vi "EXTRACT-DATA-UINT32.vi"(2 "UINT32":u32, 7 "Data":u8[](array[numeric])) -> (4 "Value":u32, 8 "Min":u32, 10 "Max":u32, 15 "Inc":u32)   [LabVIEW 2011]
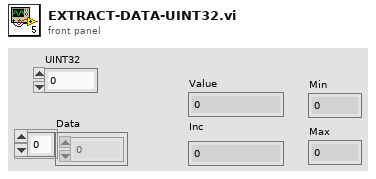
[diagram p1: front panel]
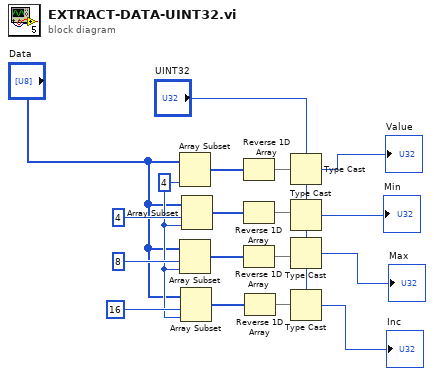
[diagram p0: block diagram]
diagram:
  w12 = 4 ("length")
  n1 = Array Subset(array="Data", length=w12) -> (w16:u8[])  [unwired: 1 in]
  n2 = Array Subset(array="Data", index=8, length=w12) -> (w17:u8[])
  n3 = Array Subset(array="Data", index=16, length=w12) -> (w11:u8[])
  n4 = Array Subset(array="Data", index=4, length=w12) -> (w18:u8[])
  n5 = Reverse 1D Array(array=w16) -> (reversed array=w10:u8[])
  n6 = Reverse 1D Array(array=w18) -> (reversed array=w9:u8[])
  n7 = Reverse 1D Array(array=w17) -> (reversed array=w8:u8[])
  n8 = Reverse 1D Array(array=w11) -> (reversed array=w7:u8[])
  n9 = Type Cast(type="UINT32", x=w10) -> (*(type *) &x=→"Value":u32)
  n10 = Type Cast(type="UINT32", x=w9) -> (*(type *) &x=→"Min":u32)
  n11 = Type Cast(type="UINT32", x=w8) -> (*(type *) &x=→"Max":u32)
  n12 = Type Cast(type="UINT32", x=w7) -> (*(type *) &x=→"Inc":u32)
